vi "String to Variant.vi"(8 "error in (no error)":errorcluster, 10 "String":string, 11 "Integer Value in":refnum<class "Integer Value.lvclass">) -> (0 "error out":errorcluster, 2 "Variant":variant, 3 "Integer Value out":refnum<class "Integer Value.lvclass">)   [LabVIEW 2020, in "Composed Columns.lvlib" / "Integer Value.lvclass"]
uses:
  Integer Value.lvclass
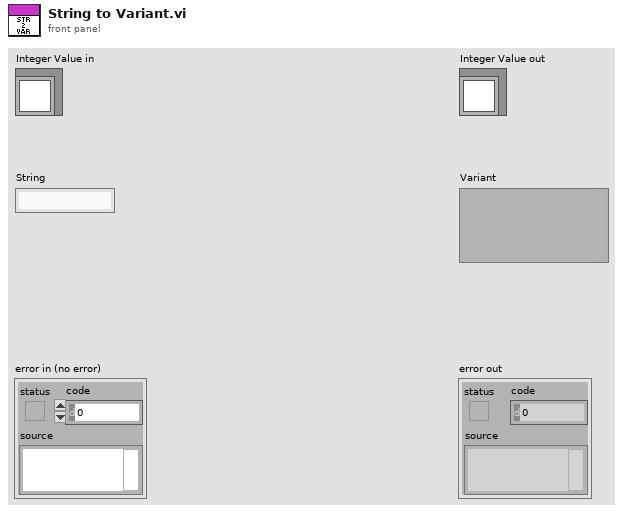
[diagram p1: front panel]
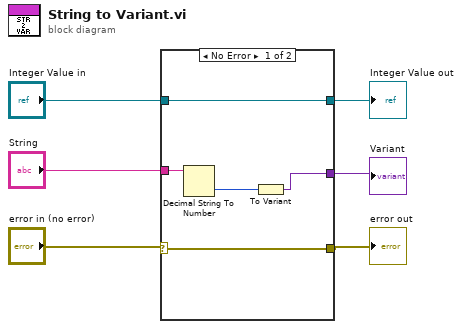
[diagram p0: block diagram]
diagram:
  n1 = case shown="No Error" "error in (no error)" {
    selector: "error in (no error)" -> [w9 w13]
    tunnel: [w9 w13] -> w5
    tunnel: "Integer Value in" -> [w10 w12]
    tunnel: [w10 w12] -> w3
    tunnel: "String" -> [w7 _]
    tunnel: [w11 _] -> w2
    frame No Error {
      n2 = Decimal String To Number(string=w7) -> (number=w8:i32)  [unwired: 2 in, 1 out]
      n3 = To Variant(anything=w8) -> (Variant=w11:variant)
    }
    frame Error {
    }
  }
  "error out" <- w5
  "Integer Value out" <- w3
  "Variant" <- w2
